vi "floor types for Cube round.vi"(10 "cnt":i32, 11 "Type":enum16{"Z", "I", "O", "S", "L", "J", "T", "N"}(ring)) -> (3 "Type required":enum16{"Z", "I", "O", "S", "L", "J", "T", "N"}(ring))   [LabVIEW 2018]
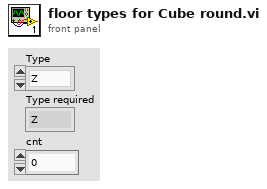
[diagram p1: front panel]
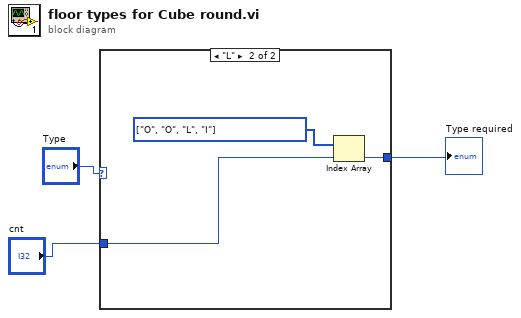
[diagram p0: block diagram]
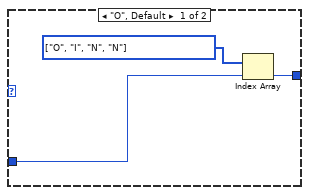
[diagram p2: hidden frame]
diagram:
  n1 = case shown="\"L\"" "Type" {
    tunnel: "cnt" -> [w5 w8]
    tunnel: [w4 w7] -> w1
    frame "O", Default {
      w6 = enum16{"Z", "I", "O", "S", "L", "J", "T", "N"}[] [enum."O", enum."I", enum."N", enum."N"] items=["Z", "I", "O", "S", "L", "J", "T", "N"] ("Type 2")
      n2 = Index Array(array=w6, index=w5) -> (element=w4:enum16{"Z", "I", "O", "S", "L", "J", "T", "N"})
    }
    frame "L" {
      w9 = enum16{"Z", "I", "O", "S", "L", "J", "T", "N"}[] [enum."O", enum."O", enum."L", enum."I"] items=["Z", "I", "O", "S", "L", "J", "T", "N"] ("Type 2")
      n3 = Index Array(array=w9, index=w8) -> (element=w7:enum16{"Z", "I", "O", "S", "L", "J", "T", "N"})
    }
  }
  "Type required" <- w1
